vi "UserVars-Edit Expression Dialog.vi"(0 "Expr In":string, 2 "Parent VI":refnum<vi>, 7 "Prompt":string="Expression") -> (4 "Expr Out":string, 8 "Canceled?":bool)   [LabVIEW 2020]
panel:
  in  "String":string caption="Expression"
  out "exit signal":bool
  in  "Cancel":bool
  in  "OK":bool
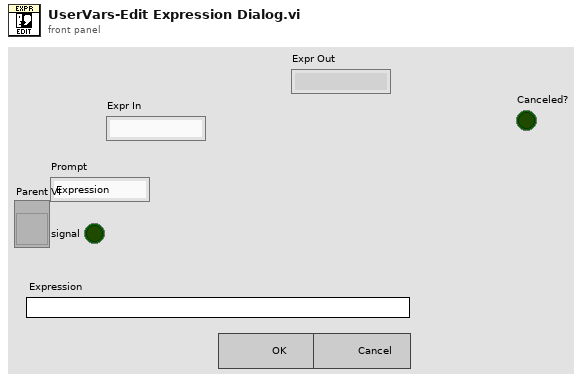
[diagram p1: front panel]
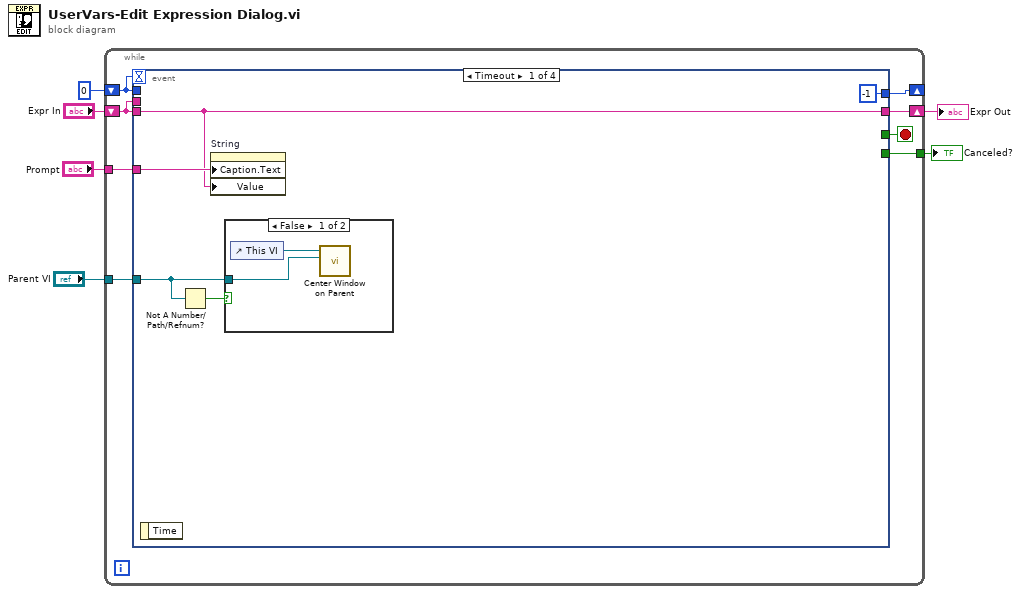
[diagram p0: block diagram]
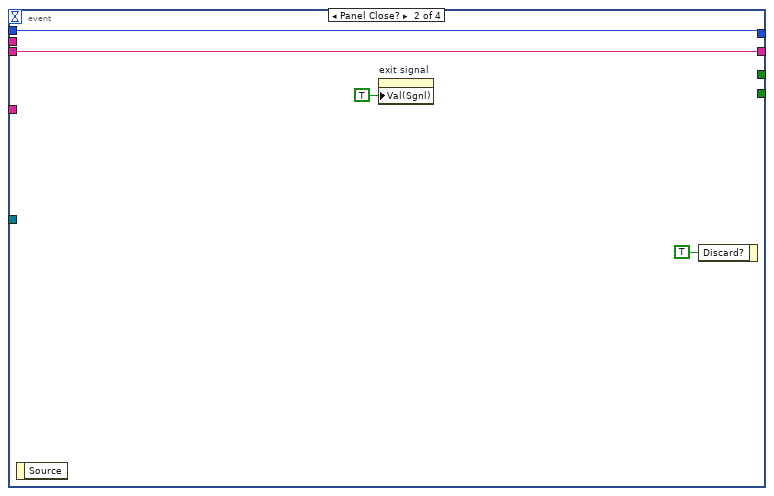
[diagram p3: hidden frame]
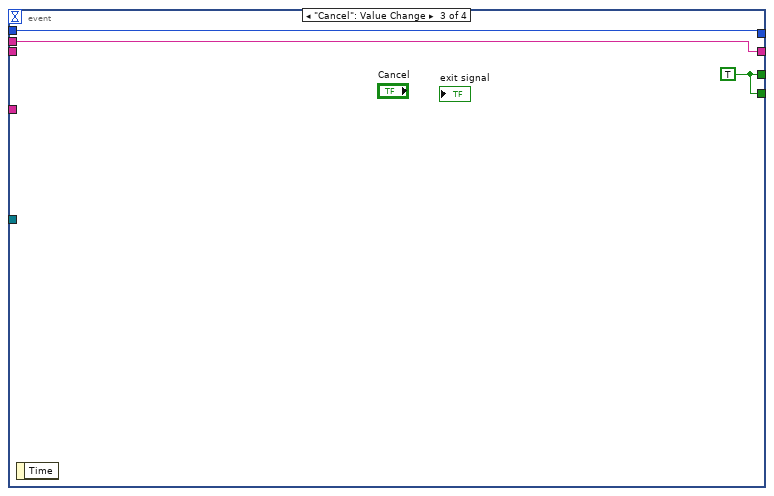
[diagram p4: hidden frame]
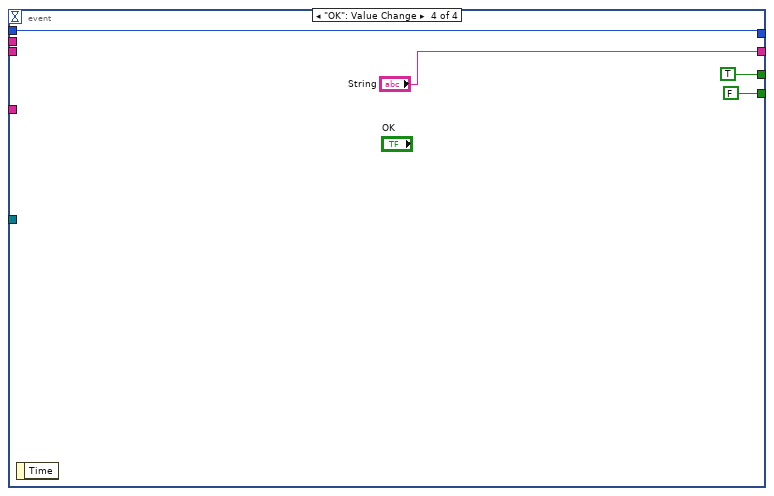
[diagram p5: hidden frame]
diagram:
  n1 = while {
    shift-right: [w14] -> _
    shift-left: 0 -> [w9]
    tunnel: [w11] -> w3
    shift-right: [w13] -> w4
    shift-left: "Expr In" -> [w10]
    tunnel: "Prompt" -> [w8]
    tunnel: "Parent VI" -> [w7]
    stop <- w12 stop-if-true
    n2 = event shown="[0] Timeout" {
      selector: _ -> [_ _ _ _]
      dyn-events: _ -> [_ _ _ _]
      timeout: w9 -> [_ _ _ _]
      tunnel: [-1 w25 w26 w30] -> w14
      tunnel: w10 -> [w17 w24 _ _]
      tunnel: [w17 w24 w27 "String"] -> w13
      tunnel: [_ _ w28 TRUE] -> w12
      tunnel: [_ _ w28 FALSE] -> w11
      tunnel: w10 -> [_ _ w27 _]
      tunnel: w9 -> [_ w25 w26 w30]
      tunnel: w8 -> [w18 _ _ _]
      tunnel: w7 -> [w16 _ _ _]
      event Timeout {
        n3 = event-data() -> ()  [unwired: 1 in, 1 out]
        n4 = Not A Number/Path/Refnum?(number/path/refnum=w16) -> (NaN/Path/Refnum?=w15:bool)
        n5 = property on="String" class="Str"("Caption.Text"=w18, "Value"=w17) -> ()  [unwired: 2 in, 2 out]
        n6 = case shown="False" w15 {
          tunnel: w16 -> [w20 _]
          frame False {
            n7 = control-ref of="This VI"() -> (w21:refnum<vi>)
            n8 = call "Center Window on Parent.vi"("Parent VI"=w20, "VI in"=w21) -> ()  [unwired: 8 in, 2 out]
          }
          frame True {
          }
        }
      }
      event Panel Close? {
        n9 = event-data() -> ()  [unwired: 1 in, 1 out]
        n10 = property on="exit signal" class="Bool (strict)"("Val(Sgnl)"=TRUE ("Value (Signaling)")) -> ()  [unwired: 2 in, 2 out]
        n11 = event-data("Discard?"=TRUE) -> ()  [unwired: 1 in, 1 out]
      }
      event "Cancel": Value Change {
        w28 = TRUE
        n12 = event-data() -> ()  [unwired: 1 in, 1 out]
      }
      event "OK": Value Change {
        n13 = event-data() -> ()  [unwired: 1 in, 1 out]
      }
    }
  }
  "Expr Out" <- w4
  "Canceled?" <- w3
